vi "Part 2.vi"() -> ()   [LabVIEW 2021]
uses:
  98d1ecff-ea60-425a-b4b0-2124b38e3b1d.vi
  c950cb29-e169-44d7-93f3-10b71ef1ba7f.vi
  <userlib>/_OpenG.lib/string/string.llb/Convert EOLs (String)__ogtk.vi
panel:
  in  "Input":string
  out "Output":i64
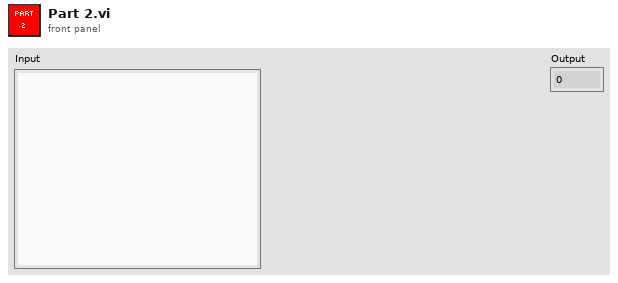
[diagram p1: front panel]
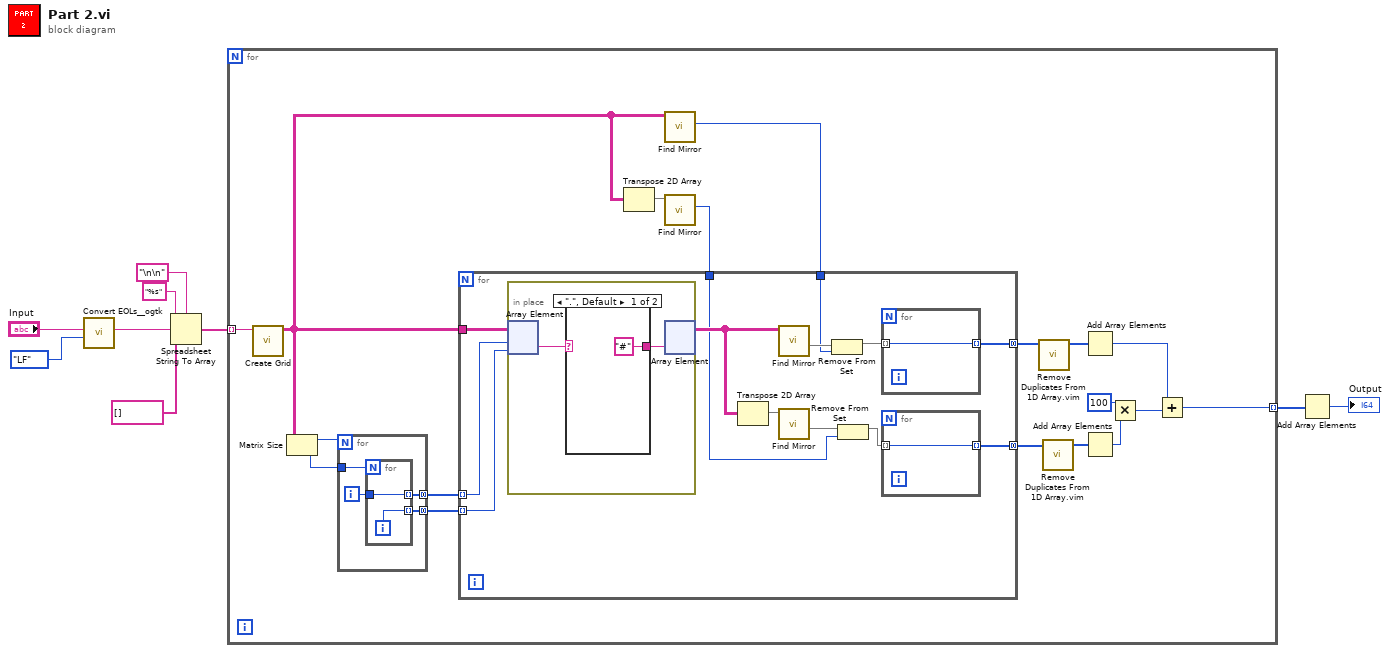
[diagram p0: block diagram]
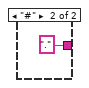
[diagram p2: hidden frame]
diagram:
  n1 = call-poly <userlib>:"Convert EOLs__ogtk.vi"("Convert to:"=enum16{"CR", "LF", "CRLF"}."LF", "String in"="Input") -> ("String out"=w5:string)  [unwired: 9 in]
  n2 = Spreadsheet String To Array(delimiter (Tab)="\n\n", format string="%s", spreadsheet string=w5, array type (2D Dbl)=string[] []) -> (array=w3:string[])
  n3 = for {
    tunnel: w3 -> [w27] mode=indexing
    tunnel: [w11] -> w1 mode=indexing
    n4 = call "Create Grid.vi"("String"=w27) -> ("Array"=w21:string[][])  [unwired: 10 in]
    n5 = Matrix Size(0:w21) -> (1:w26:i32, 2:w25:i32)
    n6 = for {
      N: w26 -> [_]
      tunnel: w25 -> [w50]
      tunnel: [w48] -> w24 mode=concatenating
      tunnel: [w47] -> w23 mode=concatenating
      i -> [w49]
      n7 = for {
        N: w50 -> [_]
        tunnel: [w52] -> w48 mode=indexing
        tunnel: w49 -> [w52]
        tunnel: [w51] -> w47 mode=indexing
        i -> [w51]
      }
    }
    n8 = Transpose 2D Array(2D array=w21) -> (transposed array=w22:string[][])
    n9 = call "Find Mirror.vi"("Array in"=w21) -> ("element"=w20:i32)  [unwired: 8 in, 2 out]
    n10 = call "Find Mirror.vi"("Array in"=w22) -> ("element"=w19:i32)  [unwired: 8 in, 2 out]
    n11 = for {
      tunnel: w21 -> [w39]
      tunnel: w24 -> [w37] mode=indexing
      tunnel: w23 -> [w36] mode=indexing
      tunnel: w20 -> [w34]
      tunnel: w19 -> [w32]
      tunnel: [w29] -> w18 mode=concatenating
      tunnel: [w28] -> w17 mode=concatenating
      n12 = in-place {
        n13 = in-place-array #1(w39, w37, w36) -> (w44:string)
        n14 = case shown="\".\", Default" w44 {
          tunnel: ["#" "."] -> w43
          frame ".", Default {
          }
          frame "#" {
          }
        }
        n15 = in-place-array #1(w43) -> (w38:string[][])  [unwired: 2 out]
      }
      n16 = Transpose 2D Array(2D array=w38) -> (transposed array=w40:string[][])
      n17 = call "Find Mirror.vi"("Array in"=w38) -> ("set"=w35:set{i32})  [unwired: 8 in, 2 out]
      n18 = call "Find Mirror.vi"("Array in"=w40) -> ("set"=w33:set{i32})  [unwired: 8 in, 2 out]
      n19 = Remove From Set(10:w34, 11:w35) -> (3:w31:set{i32})  [unwired: 1 out]
      n20 = Remove From Set(10:w32, 11:w33) -> (3:w30:set{i32})  [unwired: 1 out]
      n21 = for {
        tunnel: w31 -> [w42] mode=indexing
        tunnel: [w42] -> w29 mode=indexing
      }
      n22 = for {
        tunnel: w30 -> [w41] mode=indexing
        tunnel: [w41] -> w28 mode=indexing
      }
    }
    n23 = call "Remove Duplicates From 1D Array.vim"("array"=w18) -> ("array with duplicates removed"=w13:i32[])  [unwired: 10 in]
    n24 = call "Remove Duplicates From 1D Array.vim"("array"=w17) -> ("array with duplicates removed"=w14:i32[])  [unwired: 10 in]
    n25 = Add Array Elements(numeric array=w13) -> (sum=w12:i32)
    n26 = Add Array Elements(numeric array=w14) -> (sum=w10:i32)
    n27 = Multiply(x=100, y=w10) -> (x*y=w16:i32)
    n28 = Add(x=w12, y=w16) -> (x+y=w11:i32)
  }
  n29 = Add Array Elements(numeric array=w1) -> (sum=→"Output":i32)
